vi "Workshop Exercise 1 Solution.vi"() -> ()   [LabVIEW 2019]
uses:
  #cluster_ProductLabel.ctl
  <vilib>/Utility/config.llb/Read Key (String).vi
  <vilib>/Utility/config.llb/Read Key (U32).vi
  <vilib>/Utility/config.llb/Read Key (Double).vi
  <vilib>/Utility/config.llb/NI_LVConfig.lvlib
panel:
  out "Available Products":T1[](array[typedef])
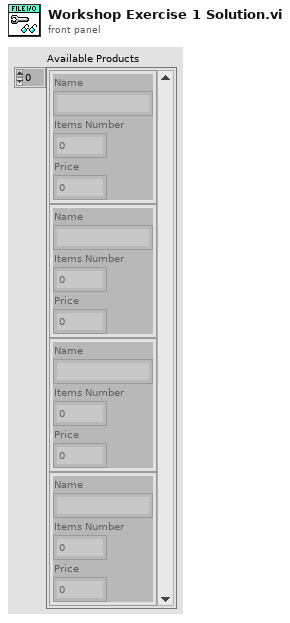
[diagram p1: front panel]
types:
  T1 = typedef "#cluster_ProductLabel.ctl" = cluster{"Name":string, "Items Number":u32, "Price":dbl}
  T2 = typedef "NI_LVConfig.lvlib/Config Data RefNum.ctl" = refnum<k1>
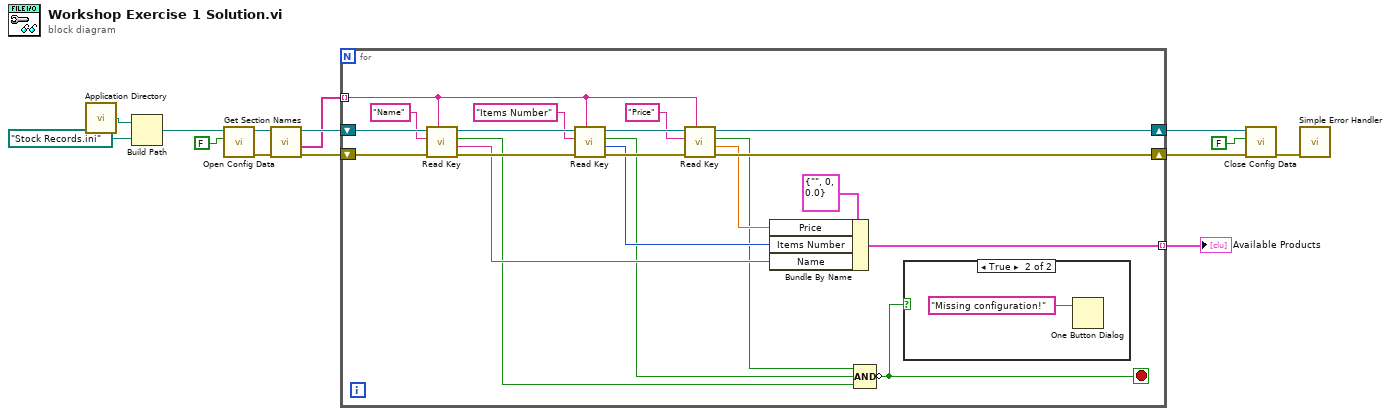
[diagram p0: block diagram]
diagram:
  n1 = call <vilib>:"Application Directory.vi"() -> ("Application Directory"=w6:path)
  n2 = Build Path(base path=w6, name or relative path=path "Stock Records.ini" ("default name")) -> (appended path=w7:path)
  n3 = call <vilib>:"Open Config Data.vi"("create file if necessary (T)"=FALSE ("create file if necessary? (T)"), "configuration file path"=w7) -> ("error out"=w12:errorcluster, "refnum"=w4:T2)  [unwired: 7 in, 1 out]
  n4 = call <vilib>:"Get Section Names.vi"("error in (no error)"=w12, "refnum"=w4) -> ("error out"=w5:errorcluster, "section names"=w2:string[], "refnum out"=w3:T2)  [unwired: 7 in]
  n5 = for {
    shift-right: [w34] -> w14
    shift-left: w5 -> [w29]
    shift-right: [w32] -> w13
    shift-left: w3 -> [w28]
    tunnel: w2 -> [w27] mode=indexing
    tunnel: [w19] -> w1 mode=indexing
    stop <- w15 stop-if-true
    n6 = call-poly <vilib>:"Read Key.vi"("section"=w27, "error in (no error)"=w29, "key"="Name", "refnum"=w28) -> ("error out"=w35:errorcluster, "value"=w22:string, "found?"=w16:bool, "refnum out"=w33:T2)  [unwired: 2 in, 2 out]
    n7 = call-poly <vilib>:"Read Key.vi"("section"=w27, "error in (no error)"=w35, "key"="Items Number", "refnum"=w33) -> ("error out"=w30:errorcluster, "value"=w21:u32, "found?"=w17:bool, "refnum out"=w31:T2)  [unwired: 1 in, 3 out]
    n8 = call-poly <vilib>:"Read Key.vi"("section"=w27, "error in (no error)"=w30, "key"="Price", "refnum"=w31) -> ("error out"=w34:errorcluster, "value"=w20:dbl, "found?"=w18:bool, "refnum out"=w32:T2)  [unwired: 1 in, 3 out]
    n9 = Bundle By Name(cluster=T1 {"Name"="", "Items Number"=0, "Price"=0.0} ("input cluster"), "Price"=w20, "Items Number"=w21, "Name"=w22) -> (w19:T1)
    n10 = Compound Arithmetic op=AND(w18, w17, w16) -> (invert w15:bool)
    n11 = case shown="True" w15 {
      frame False {
      }
      frame True {
        n12 = One Button Dialog(message="Missing configuration!") -> ()  [unwired: 1 in, 1 out]
      }
    }
  }
  "Available Products" <- w1
  n13 = call <vilib>:"Close Config Data.vi"("error in (no error)"=w14, "write file if changed (T)"=FALSE ("write configuration file? (T)"), "refnum"=w13) -> ("error out"=w9:errorcluster)  [unwired: 8 out]
  n14 = call <vilib>:"Simple Error Handler.vi"("error in (no error)"=w9) -> ()  [unwired: 1 in, 8 out]
